vi "UI_Initialize.vi"(8 "error in (no error)":errorcluster, 11 "DAQ_Module in":refnum<class "DAQ_Module.lvclass">) -> (0 "error out":errorcluster, 3 "DAQ_Module out":refnum<class "DAQ_Module.lvclass">)   [LabVIEW 2025, in "DAQ_Module.lvlib" / "DAQ_Module.lvclass"]
uses:
  DAQ_Module.lvclass
  DAQ_Module.lvclass/DAQ_Module.ctl
  <vilib>/Test Bench Framework/Client Message(Context).vi
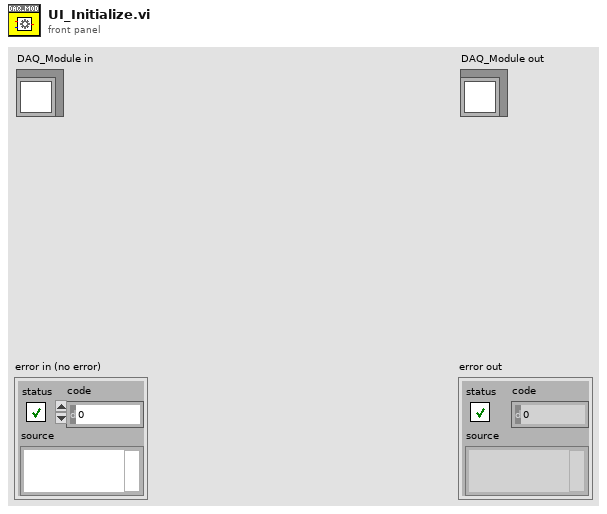
[diagram p1: front panel]
types:
  T1 = cluster{"ModelName":string, "This VI":refnum<vi>}
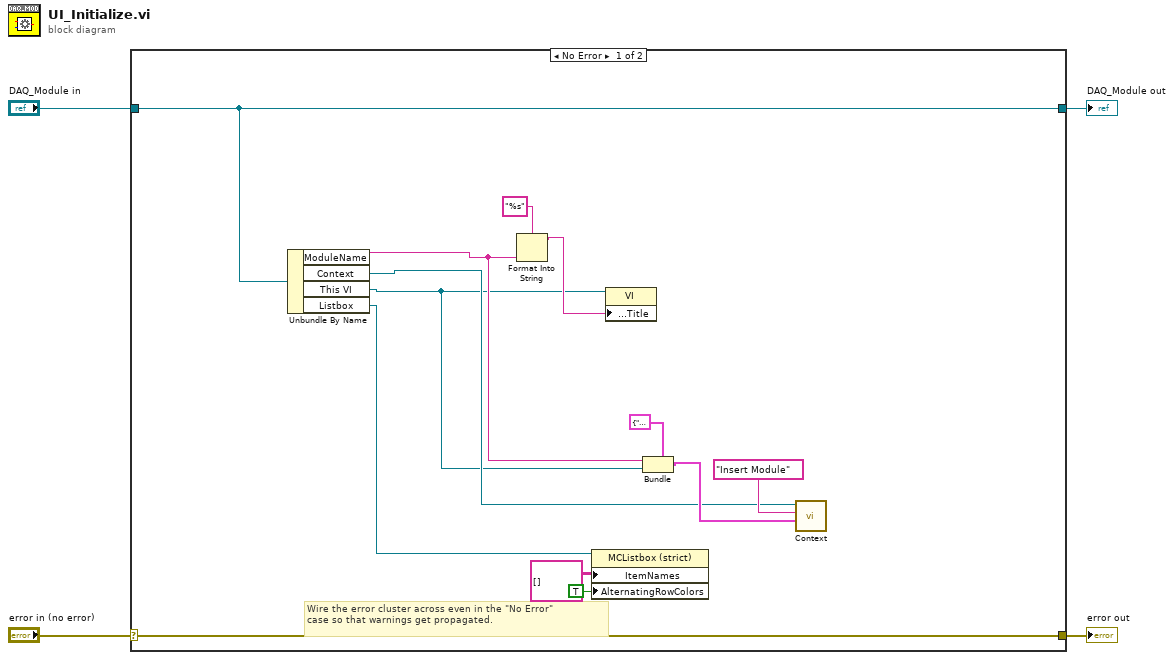
[diagram p0: block diagram]
diagram:
  n1 = case shown="No Error" "error in (no error)" {
    selector: "error in (no error)" -> [w17 w19]
    tunnel: [w17 w19] -> w3
    tunnel: [w9 w18] -> w1
    tunnel: "DAQ_Module in" -> [w9 w18]
    frame No Error {
      # "Wire the error cluster across even in the \"No Error\"\ncase so that warnings get propagated."
      n2 = Unbundle By Name(w9) -> ("ModuleName"=w10:string, "Context"=w11:refnum<vi>, "This VI"=w8:refnum<vi>, "Listbox"=w7:refnum<vi>)
      n3 = Format Into String(format string="%s", w10) -> (resulting string=w15:string)  [unwired: 2 in, 1 out]
      n4 = property class="MCListbox (strict)"(reference=w7, "ItemNames"=string[][] [] ("Item Names"), "AlternatingRowColors"=TRUE ("Alternating Row Colors")) -> ()  [unwired: 1 in, 2 out]
      n5 = property class="VI"(reference=w8, "Front Panel.Title"=w15) -> ()  [unwired: 1 in, 2 out]
      n6 = Bundle(cluster=T1 {"ModelName"="", "This VI"=refnum}, "ModelName"=w10, "This VI"=w8) -> (w14:T1)
      n7 = call-poly <vilib>:"Context.vi"("Value"=w14, "Msg"="Insert Module", "Context"=w11) -> ()  [unwired: 8 in, 1 out]
    }
    frame Error {
    }
  }
  "error out" <- w3
  "DAQ_Module out" <- w1
